vi "Mirror_Up_Down_Strings.vi"() -> (0 "Mirror Down":string="_Mirror_Down.stl", 1 "Mirror Up":string="_Mirror_Up.stl")   [LabVIEW 2022 SP3]
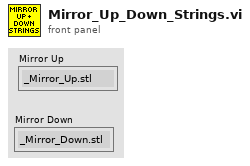
[diagram p1: front panel]
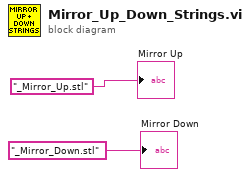
[diagram p0: block diagram]
diagram:
  "Mirror Up" <- "_Mirror_Up.stl"
  "Mirror Down" <- "_Mirror_Down.stl"
